vi "pumpy.vi"(0 "Serial port":string="COM1", 1 "Address":i32, 2 "Wait for target":bool, 3 "Syringe diameter (mm)":i32, 4 "Flow rate (uL/min)":i32, 5 "PHD2000":bool, 8 "Target volume (uL)":i32, 9 "State":u16(ring)=3 items=["Infuse", "Withdraw", "Stop", "Do nothing"]) -> (7 "output":string)   [LabVIEW 2013]
panel:
  out "command":string
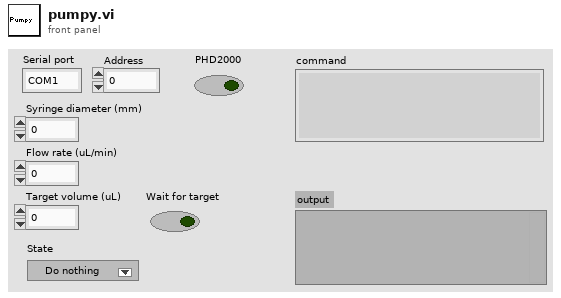
[diagram p1: front panel]
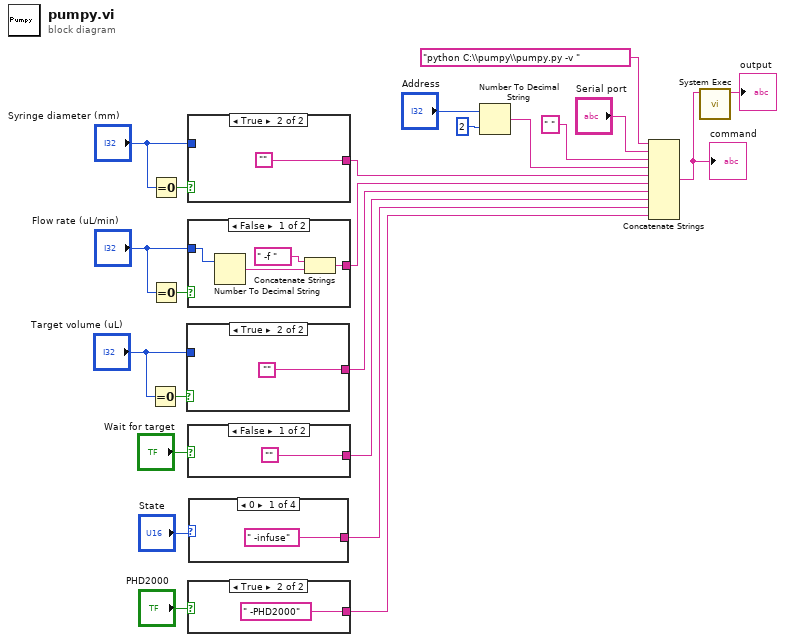
[diagram p0: block diagram]
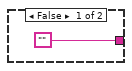
[diagram p2: hidden frame]
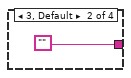
[diagram p3: hidden frame]
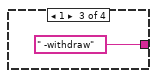
[diagram p4: hidden frame]
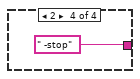
[diagram p5: hidden frame]
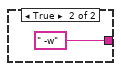
[diagram p6: hidden frame]
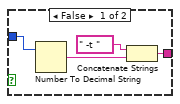
[diagram p7: hidden frame]
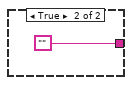
[diagram p8: hidden frame]
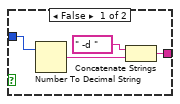
[diagram p9: hidden frame]
diagram:
  n1 = Equal To 0?(x="Target volume (uL)") -> (x = 0?=w11:bool)
  n2 = Equal To 0?(x="Syringe diameter (mm)") -> (x = 0?=w15:bool)
  n3 = Equal To 0?(x="Flow rate (uL/min)") -> (x = 0?=w13:bool)
  n4 = case shown="True" w11 {
    tunnel: "Target volume (uL)" -> [w25 _]
    tunnel: [w24 ""] -> w7
    frame False {
      n5 = Number To Decimal String(number=w25) -> (decimal integer string=w26:string)  [unwired: 1 in]
      n6 = Concatenate Strings(" -t " ("string"), w26) -> (w24:string)
    }
    frame True {
    }
  }
  n7 = case shown="True" w15 {
    tunnel: "Syringe diameter (mm)" -> [w30 _]
    tunnel: [w29 ""] -> w9
    frame False {
      n8 = Number To Decimal String(number=w30) -> (decimal integer string=w31:string)  [unwired: 1 in]
      n9 = Concatenate Strings(" -d " ("string"), w31) -> (w29:string)
    }
    frame True {
    }
  }
  n10 = case shown="False" w13 {
    tunnel: "Flow rate (uL/min)" -> [w35 _]
    tunnel: [w34 ""] -> w8
    frame False {
      n11 = Number To Decimal String(number=w35) -> (decimal integer string=w36:string)  [unwired: 1 in]
      n12 = Concatenate Strings(" -f " ("string"), w36) -> (w34:string)
    }
    frame True {
    }
  }
  n13 = case shown="False" "Wait for target" {
    tunnel: ["" " -w"] -> w5
    frame False {
    }
    frame True {
    }
  }
  n14 = case shown="True" "PHD2000" {
    tunnel: ["" " -PHD2000"] -> w1
    frame False {
    }
    frame True {
    }
  }
  n15 = case shown="0" "State" {
    tunnel: [" -infuse" "" " -withdraw" " -stop"] -> w3
    frame 0 {
    }
    frame 3, Default {
    }
    frame 1 {
    }
    frame 2 {
    }
  }
  n16 = Number To Decimal String(number="Address", width (-)=i16 2) -> (decimal integer string=w16:string)
  n17 = Concatenate Strings("python C:\\pumpy\\pumpy.py -v " ("command line"), "Serial port", " " ("string"), w16, w9, w8, w7, w5, w3, w1) -> (w22:string)
  "command" <- w22
  n18 = call <vilib>:"System Exec.vi"("command line"=w22) -> ("standard output"=→"output":string)  [unwired: 7 in, 3 out]
